vi "PushBackgate.vi"(6 "StartTime":timestamp, 8 "reference":refnum<vi>, 11 "Array":string[](array[string])) -> (0 "Current Time":dbl, 1 "Backgate":bool, 2 "Style":u16(ring) items=["Ramp+-", "Pos-Neg", "Ramp"], 3 "Enqueue":string, 4 "Range (+-) (V)":dbl=60.0 min=1.0 max=60.0)   [LabVIEW 2019, in "Scripts.lvclass"]
uses:
  Scripts.lvclass
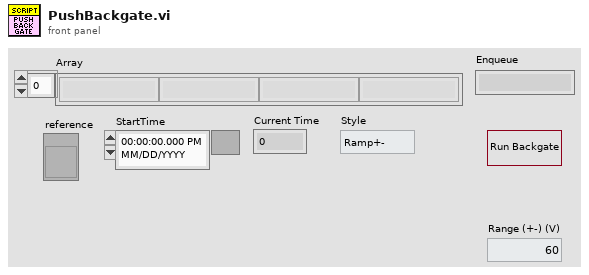
[diagram p1: front panel]
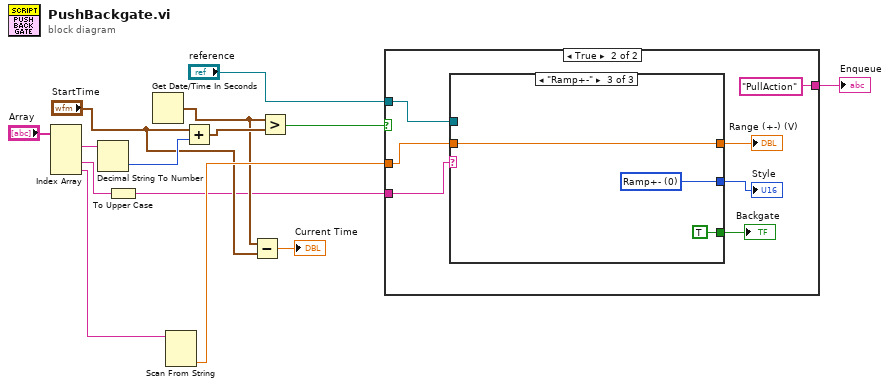
[diagram p0: block diagram]
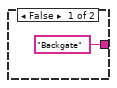
[diagram p2: hidden frame]
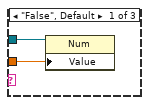
[diagram p3: hidden frame]
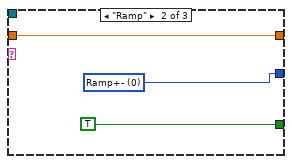
[diagram p4: hidden frame]
diagram:
  n1 = Index Array(array="Array") -> (element #1=w13:string, element #3=w3:string, element #4=w1:string)  [unwired: 4 in, 1 out]
  n2 = Decimal String To Number(string=w13) -> (number=w12:i32)  [unwired: 2 in, 1 out]
  n3 = To Upper Case(1:w3) -> (0:w2:string)
  n4 = Get Date/Time In Seconds() -> (seconds since 1Jan1904=w5:timestamp)
  n5 = Scan From String(input string=w1) -> (output 1=w8:dbl)  [unwired: 4 in, 3 out]
  n6 = Add(x="StartTime", y=w12) -> (x+y=w7:timestamp)
  n7 = Subtract(x=w5, y="StartTime") -> (x-y=→"Current Time":dbl)
  n8 = Greater?(x=w5, y=w7) -> (0:w11:bool)
  n9 = case shown="True" w11 {
    tunnel: w8 -> [_ w20]
    tunnel: ["Backgate" ("element") "PullAction" ("element")] -> w10
    tunnel: "reference" -> [_ w21]
    tunnel: w2 -> [_ w19]
    frame False {
    }
    frame True {
      n10 = case shown="\"Ramp+-\"" w19 {
        tunnel: w21 -> [w24 _ _]
        tunnel: w20 -> [w23 w27 w30]
        tunnel: [_ w27 w30] -> w18
        tunnel: [_ TRUE TRUE] -> w17
        tunnel: [_ w25 w29] -> w16
        frame "False", Default {
          n11 = property class="Num"(reference=w24, "Value"=w23) -> ()  [unwired: 1 in, 2 out]
        }
        frame "Ramp" {
          w25 = u16 0 items=["Ramp+-", "Pos-Neg", "Ramp"] ("Style")
        }
        frame "Ramp+-" {
          w29 = u16 0 items=["Ramp+-", "Pos-Neg", "Ramp"] ("Style")
        }
      }
      "Range (+-) (V)" <- w18
      "Style" <- w16
      "Backgate" <- w17
    }
  }
  "Enqueue" <- w10
